vi "load_kbolott_volume.vi"() -> (0 "output":dbl[][](array[numeric]))   [LabVIEW 2014]
uses:
  <vilib>/Analysis/Matrix/Datatypes/RealMatrix.ctl
  <vilib>/Utility/file.llb/Read From Spreadsheet File (DBL).vi
  <vilib>/Utility/file.llb/Write To Spreadsheet File (DBL).vi
  <vilib>/Analysis/Matrix/NI_Matrix.lvlib
panel:
  out "Path":path
  in  "Diagnostics PC?":bool=TRUE
  in  "DEBUG AT 1-4":string="6"
  out "TMP":T1
  in  "DEBUG":bool=TRUE
  out "VBCr Import":T1
  out "VBCl Import (0-16)":T1
  out "VBCl Import (17-24)":T1
  out "HBCm Import":T1
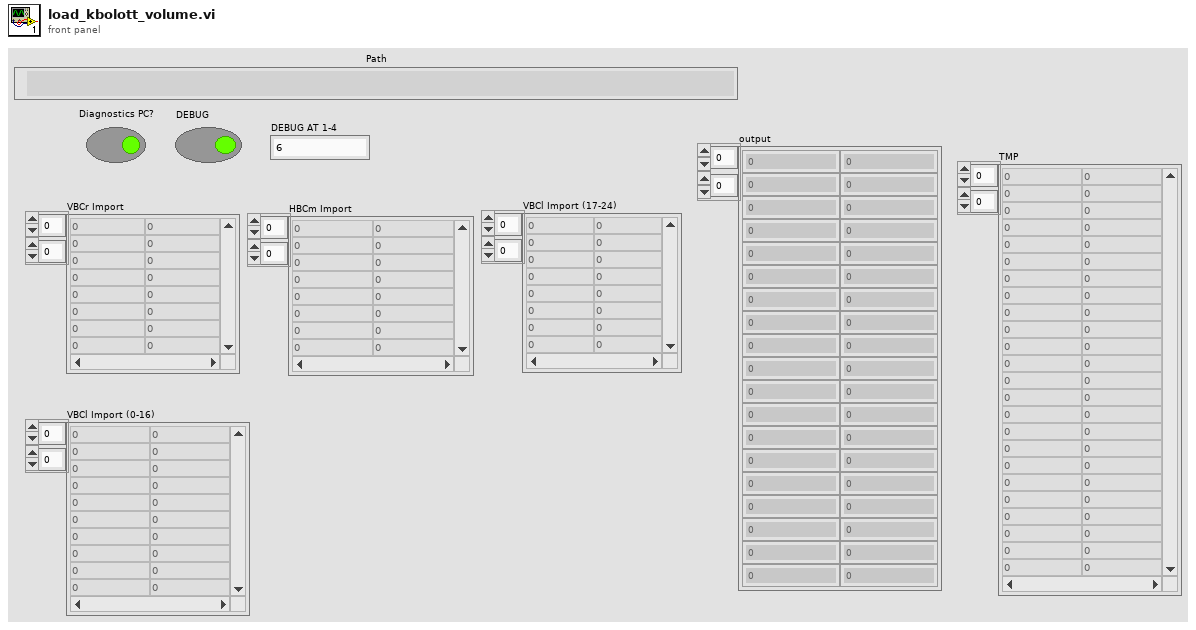
[diagram p1: front panel]
types:
  T1 = typedef "NI_Matrix.lvlib/RealMatrix.ctl" = dbl[][]
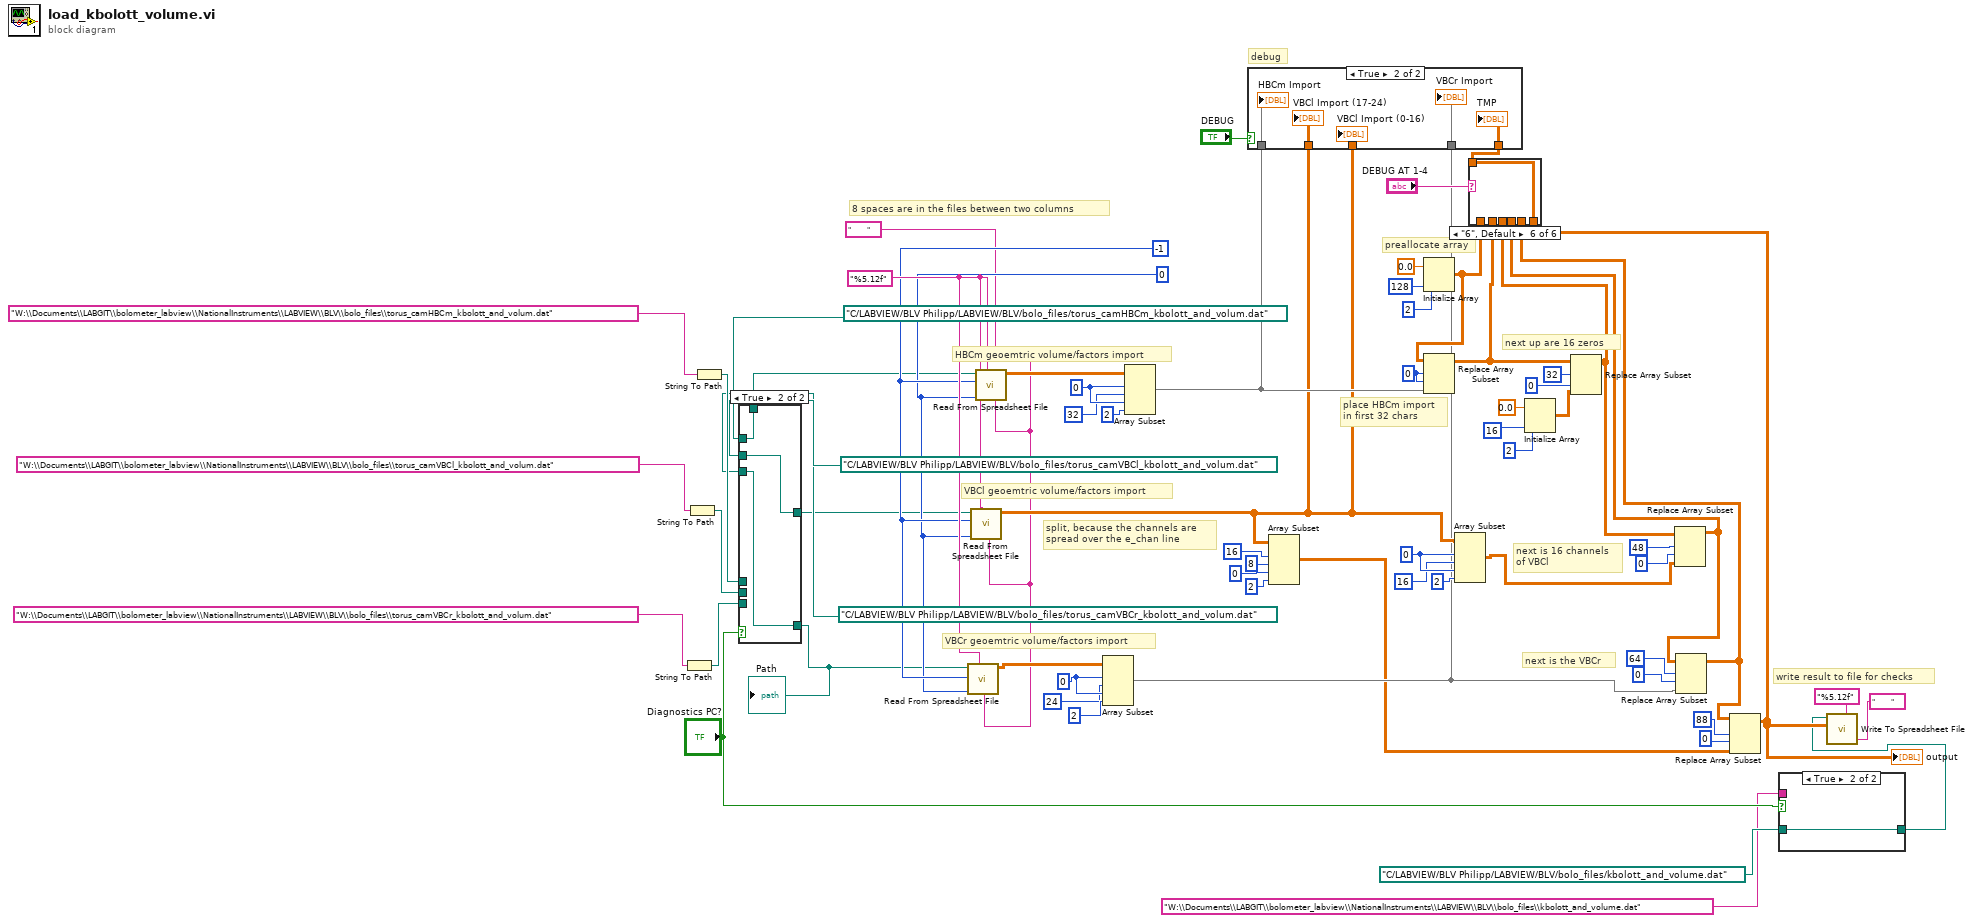
[diagram p0: block diagram]
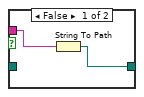
[diagram p2: hidden frame]
diagram:
  w46 = 0 ("index (row)")
  w52 = 0
  w60 = 0
  w67 = 0
  w2 = "        "
  w55 = 0
  w57 = "%5.12f"
  w56 = -1
  # "write result to file for checks"
  # "next is the VBCr"
  # "next is 16 channels\nof VBCl"
  # "next up are 16 zeros"
  # "place HBCm import\nin first 32 chars"
  # "preallocate array"
  # "split, because the channels are\nspread over the e_chan line"
  # "VBCr geoemtric volume/factors import"
  # "VBCl geoemtric volume/factors import"
  # "HBCm geoemtric volume/factors import"
  # "debug"
  # "8 spaces are in the files between two columns"
  n1 = String To Path(string="W:\\Documents\\LABGIT\\bolometer_labview\\NationalInstruments\\LABVIEW\\BLV\\bolo_files\\torus_camVBCr_kbolott_and_volum.dat") -> (path=w8:path)
  n2 = String To Path(string="W:\\Documents\\LABGIT\\bolometer_labview\\NationalInstruments\\LABVIEW\\BLV\\bolo_files\\torus_camVBCl_kbolott_and_volum.dat") -> (path=w15:path)
  n3 = String To Path(string="W:\\Documents\\LABGIT\\bolometer_labview\\NationalInstruments\\LABVIEW\\BLV\\bolo_files\\torus_camHBCm_kbolott_and_volum.dat") -> (path=w16:path)
  n4 = case shown="True" "Diagnostics PC?" {
    tunnel: w16 -> [w68 _]
    tunnel: w15 -> [w69 _]
    tunnel: w8 -> [w70 _]
    tunnel: path "C:/LABVIEW/BLV Philipp/LABVIEW/BLV/bolo_files/torus_camHBCm_kbolott_and_volum.dat" -> [_ w71]
    tunnel: path "C:/LABVIEW/BLV Philipp/LABVIEW/BLV/bolo_files/torus_camVBCl_kbolott_and_volum.dat" -> [_ w72]
    tunnel: path "C:/LABVIEW/BLV Philipp/LABVIEW/BLV/bolo_files/torus_camVBCr_kbolott_and_volum.dat" -> [_ w73]
    tunnel: [w70 w73] -> w1
    tunnel: [w69 w72] -> w10
    tunnel: [w68 w71] -> w9
    frame False {
    }
    frame True {
    }
  }
  "Path" <- w1
  n5 = call-poly <vilib>:"Read From Spreadsheet File.vi"("delimiter (\\t)"=w2, "format (%.3f)"=w57, "max characters/row  (no limit:0)"=w55, "number of rows (all:-1)"=w56, "file path (dialog if empty)"=w1) -> ("all rows"=w53:dbl[][])  [unwired: 2 in, 4 out]
  n6 = call-poly <vilib>:"Read From Spreadsheet File.vi"("delimiter (\\t)"=w2, "format (%.3f)"=w57, "max characters/row  (no limit:0)"=w55, "number of rows (all:-1)"=w56, "file path (dialog if empty)"=w10) -> ("all rows"=w37:dbl[][])  [unwired: 2 in, 4 out]
  n7 = call-poly <vilib>:"Read From Spreadsheet File.vi"("delimiter (\\t)"=w2, "format (%.3f)"=w57, "max characters/row  (no limit:0)"=w55, "number of rows (all:-1)"=w56, "file path (dialog if empty)"=w9) -> ("all rows"=w54:dbl[][])  [unwired: 2 in, 4 out]
  n8 = Array Subset(array=w53, index (row)=w52, length (row)=24, index (col)=w52, length (col)=2) -> (w29:dbl[][])
  n9 = Array Subset(array=w54, index (row)=w60, length (row)=32, index (col)=w60, length (col)=2) -> (w38:dbl[][])
  n10 = Array Subset(array=w37, index (row)=16, length (row)=8, index (col)=0, length (col)=2) -> (w23:dbl[][])
  n11 = Initialize Array(0.0 ("element"), 128 ("dimension size"), 2 ("dimension size")) -> (w34:dbl[][])
  n12 = Replace Array Subset(array=w34, new element=w38, index (row)=w46, index (col)=w46) -> (w32:dbl[][])
  n13 = Array Subset(array=w37, index (row)=w67, length (row)=16, index (col)=w67, length (col)=2) -> (w30:dbl[][])
  n14 = Initialize Array(0.0 ("element"), 16 ("dimension size"), 2 ("dimension size")) -> (w35:dbl[][])
  n15 = Replace Array Subset(array=w32, new element=w35, index (row)=32, index (col)=0 ("disabled index (col)")) -> (w26:dbl[][])
  n16 = Replace Array Subset(array=w26, new element=w30, index (row)=48, index (col)=0 ("disabled index (col)")) -> (w25:dbl[][])
  n17 = Replace Array Subset(array=w25, new element=w29, index (row)=64, index (col)=0 ("disabled index (col)")) -> (w24:dbl[][])
  n18 = Replace Array Subset(array=w24, new element=w23, index (row)=88, index (col)=0 ("disabled index (col)")) -> (w19:dbl[][])
  "output" <- w19
  n19 = case shown="\"6\", Default" "DEBUG AT 1-4" {
    tunnel: w34 -> [w74 _ _ _ _ _]
    tunnel: [w74 w75 w76 w77 w78 w79] -> w33
    tunnel: w32 -> [_ w75 _ _ _ _]
    tunnel: w26 -> [_ _ w76 _ _ _]
    tunnel: w25 -> [_ _ _ w77 _ _]
    tunnel: w24 -> [_ _ _ _ w78 _]
    tunnel: w19 -> [_ _ _ _ _ w79]
    frame "1" {
    }
    frame "2" {
    }
    frame "3" {
    }
    frame "4" {
    }
    frame "5" {
    }
    frame "6", Default {
    }
  }
  n20 = case shown="True" "DEBUG" {
    tunnel: w38 -> [_ w84]
    tunnel: w37 -> [_ w83]
    tunnel: w37 -> [_ w82]
    tunnel: w29 -> [_ w81]
    tunnel: w33 -> [_ w80]
    frame False {
    }
    frame True {
      "VBCr Import" <- w81
      "HBCm Import" <- w84
      "VBCl Import (17-24)" <- w83
      "VBCl Import (0-16)" <- w82
      "TMP" <- w80
    }
  }
  n21 = case shown="True" "Diagnostics PC?" {
    tunnel: path "C:/LABVIEW/BLV Philipp/LABVIEW/BLV/bolo_files/kbolott_and_volume.dat" -> [_ w87]
    tunnel: [w85 w87] -> w5
    tunnel: "W:\\Documents\\LABGIT\\bolometer_labview\\NationalInstruments\\LABVIEW\\BLV\\bolo_files\\kbolott_and_volume.dat" -> [w86 _]
    frame False {
      n22 = String To Path(string=w86) -> (path=w85:path)
    }
    frame True {
    }
  }
  n23 = call-poly <vilib>:"Write To Spreadsheet File.vi"("delimiter (\\t)"="        " ("delimiter (\\t)"), "format (%.3f)"="%5.12f", "2D data"=w19, "file path (dialog if empty)"=w5) -> ()  [unwired: 4 in, 1 out]
